vi "ziGetValue.vi"   [LabVIEW 2009, in "Zurich Instruments LabOne.lvlib"]
doc: "This polymorphic vi gets values from nodes specified by <b>Path</b>."
uses:
  <instrlib>/Zurich Instruments LabOne/Zurich Instruments LabOne.lvlib
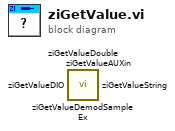
[diagram p0: block diagram]
diagram:
  n1 = call <instrlib>:"ziGetValueDemodSampleEx.vi"() -> ()  [unwired: 3 in, 3 out]
  n2 = call <instrlib>:"ziGetValueAUXin.vi"() -> ()  [unwired: 3 in, 3 out]
  n3 = call <instrlib>:"ziGetValueDIO.vi"() -> ()  [unwired: 3 in, 3 out]
  n4 = call <instrlib>:"ziGetValueString.vi"() -> ()  [unwired: 3 in, 3 out]
  n5 = call <instrlib>:"ziGetValueDouble.vi"() -> ()  [unwired: 3 in, 3 out]
